vi "pp3_cam_display.vi"(8 "Camera":T1="cam0", 9 "Log File Directory":refnum<vi>, 10 "State info Refnum":refnum<vi>, 11 "Image Ctl Refnum":refnum<vi>) -> ()   [LabVIEW 2013]
doc: "This VI is a general VI that loops through webcam images, and saves when necessary. It should be run asynchronously, so that webcam display/logging is independent of the main loop. Terminate this VI by setting the \"Webcam on\" value within the state info refnum to False."
uses:
  pp3_CTL_StateInfo.ctl
  pp3_CTL_State.ctl
  pp3_CTL_Trial.ctl
  pp3_CTL_TrialType.ctl
  labolabo2/waveforms/WFTypes.ctl
  <vilib>/userdefined/High Color/IMAQdx.ctl
  <vilib>/vision/Image Controls.llb/IMAQ Image.ctl
  <vilib>/vision/driver/NI_Vision_Acquisition_Software.lvlib
panel:
  out "error out":errorcluster
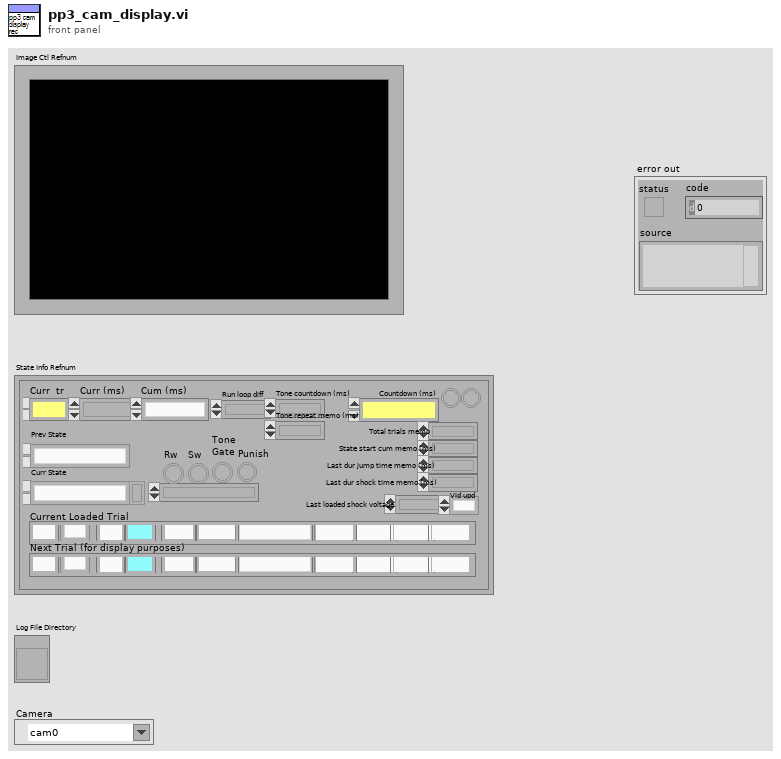
[diagram p1: front panel]
types:
  T1 = typedef "IMAQdx.ctl" = refnum<k21>
  T2 = typedef "pp3_CTL_StateInfo.ctl" = cluster{"Curr  tr":u16, "Curr (ms)":u32, "Cum (ms)":i64, "Run loop diff":i64, "Tone countdown (ms)":i64, "Countdown (ms)":i64, "Curr State":T3, "Prev State":T3, "Rw":bool, "Sw":bool, "Tone\nGate":bool, "Punish":bool, "Current DAQ DO Int":u16, "Current Loaded Trial":T4, "Next Trial (for display purposes)":T4, "Total trials memo":i64, "State start cum memo (ms)":i64, "Last dur jump time memo (ms)":i64, "Last dur shock time memo (ms)":i64, "Tone repeat memo (ms)":i64, "Webcam on":bool, "Webcam recording":bool, "State update flag":bool, "Last loaded shock voltage":dbl, "Vid upd":enum16{"0", "1", "2", "3", "4", "5", "6", "7", "8", "9"}}
  T3 = typedef "pp3_CTL_State.ctl" = enum8{"0 NULL", "1 Habituation", "2 (Load Trial)", "3 Stay Period", "4 Load Audio/Click Delay", "5 GO Trial", "6 GO Jumped", "7 GO Timeout", "8 NOGO Trial", "9 NOGO Jumped", "10 NOGO Timeout", "11 TEST Trial", "12 TEST Jumped", "13 TEST Timeout", "14 Intertrial Interval", "15 Done"}
  T4 = typedef "pp3_CTL_Trial.ctl" = cluster{"Trial Type Number":i16, "Trial Type":T5, "Trial Weight":u32, "Shock (mA)":dbl, "Duration (ms)":dbl, "Sound Type":T6, "Stim P1":dbl, "Stim P2":dbl, "Stim P3":dbl, "Stim P4":dbl, "DAQ Amplitude (V)":dbl}
  T5 = typedef "pp3_CTL_TrialType.ctl" = enum16{"OFF", "GO", "NOGO", "TEST"}
  T6 = typedef "WFTypes.ctl" = enum16{"00 NULL", "01 DC", "02 Noise", "03 Pure Tone", "04 FM Sweep"}
  T7 = typedef "IMAQ Image.ctl" = refnum<image>
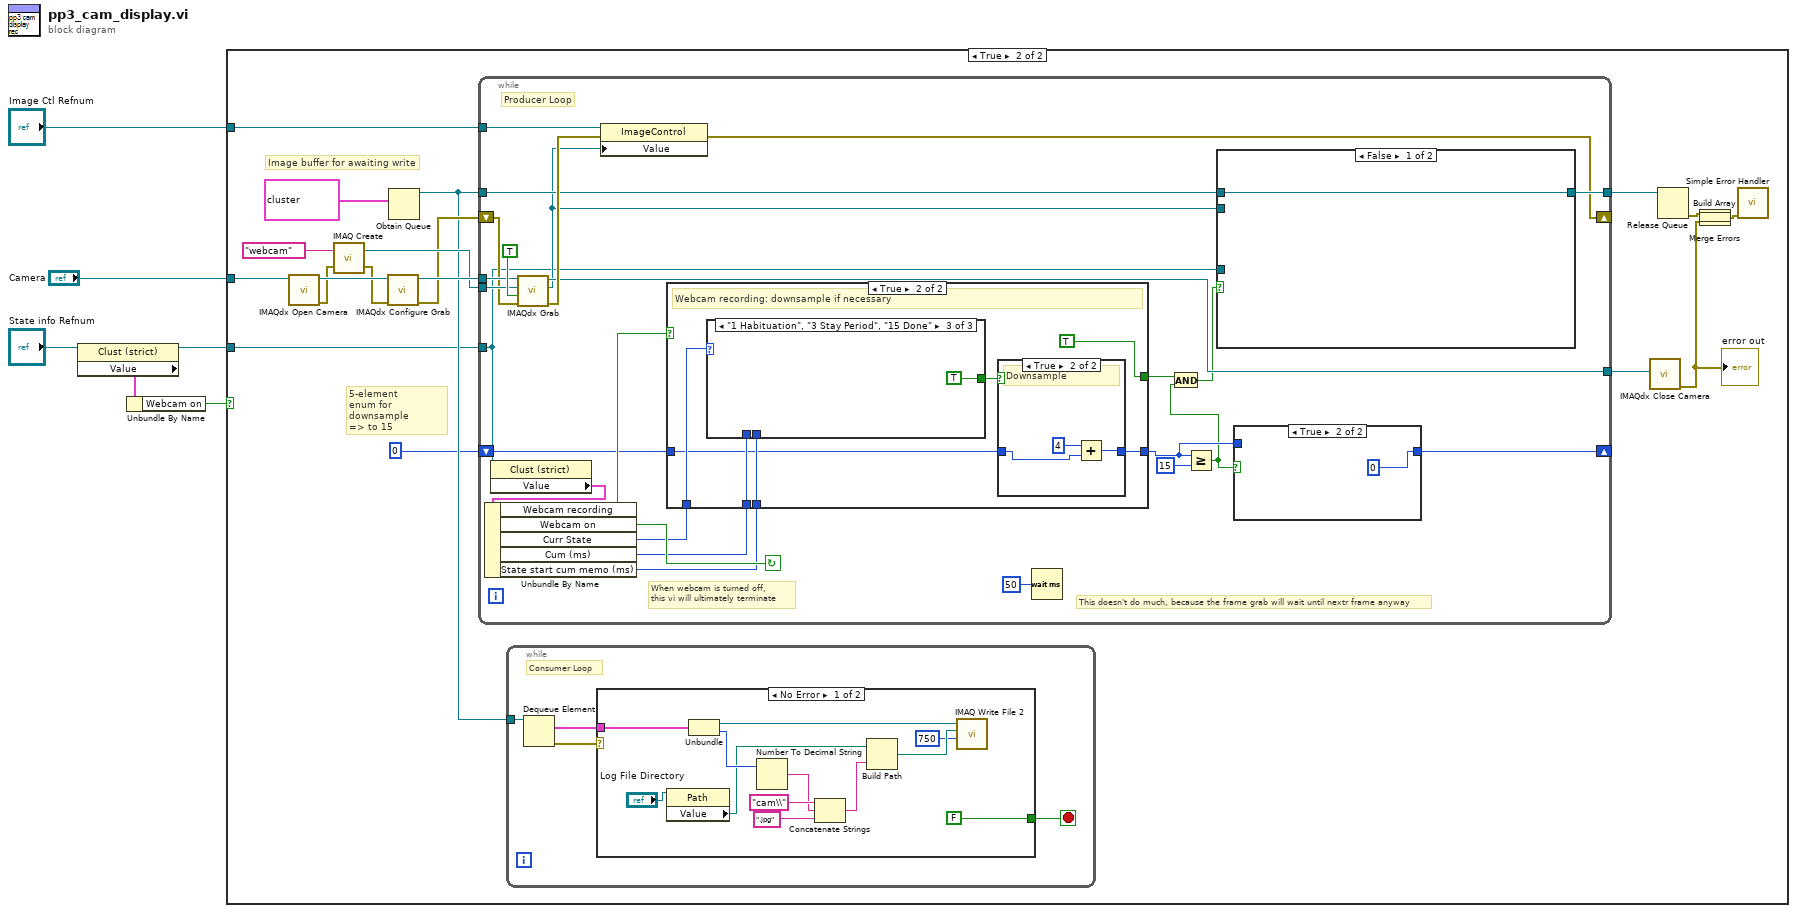
[diagram p0: block diagram]
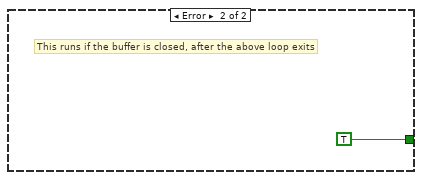
[diagram p3: hidden frame]
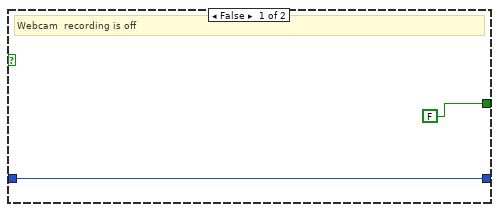
[diagram p5: hidden frame]
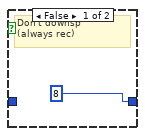
[diagram p6: hidden frame]
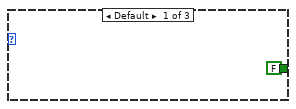
[diagram p7: hidden frame]
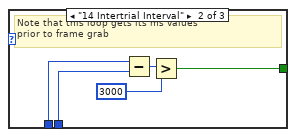
[diagram p8: hidden frame]
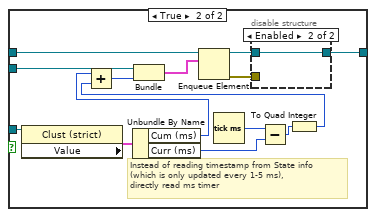
[diagram p9: hidden frame]
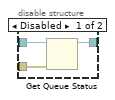
[diagram p10: hidden frame]
diagram:
  n1 = property class="Clust (strict)"(reference="State info Refnum") -> (reference out=w3:refnum<vi>, "Value"=w2:T2)  [unwired: 1 in, 1 out]
  n2 = Unbundle By Name(w2) -> ("Webcam on"=w1:bool)
  n3 = case shown="True" w1 {
    tunnel: "Image Ctl Refnum" -> [_ w25]
    tunnel: "Camera" -> [_ w21]
    tunnel: w3 -> [_ w8]
    frame False {
    }
    frame True {
      # "5-element\nenum for downsample\n=> to 15"
      # "Image buffer for awaiting write"
      n4 = call <vilib>:"IMAQdx Open Camera.vi"("Session In"=w21) -> ("error out"=w20:errorcluster, "Session Out"=w23:T1)  [unwired: 9 in]
      n5 = call "IMAQ Create"("Image Name"="webcam", "error in (no error)"=w20) -> ("New Image"=w17:T7, "error out"=w19:errorcluster)  [unwired: 3 in]
      n6 = call <vilib>:"IMAQdx Configure Grab.vi"("error in"=w19, "Session In"=w23) -> ("error out"=w11:errorcluster, "Session Out"=w18:T1)  [unwired: 8 in]
      n7 = Obtain Queue(element data type=cluster{"Image":T7, "Cum (ms)":i64} {"Image"="Webcam", "Cum (ms)"=0}) -> (queue out=w9:refnum<queue>)  [unwired: 4 in, 2 out]
      n8 = while {
        tunnel: w18 -> [w65]
        tunnel: w17 -> [w64]
        tunnel: w9 -> [w63]
        tunnel: [w61] -> w16
        tunnel: [w60] -> w12
        shift-right: [w57] -> _
        shift-left: w11 -> [w59]
        tunnel: w8 -> [w56]
        tunnel: w25 -> [w67]
        shift-right: [w48] -> _
        shift-left: 0 -> [w50]
        stop <- w62 continue-if-true
        # "This doesn't do much, because the frame grab will wait until nextr frame anyway"
        # "When webcam is turned off,\nthis vi will ultimately terminate"
        # "Producer Loop"
        n9 = property class="Clust (strict)"(reference=w56) -> ("Value"=w54:T2)  [unwired: 1 in, 2 out]
        n10 = Unbundle By Name(w54) -> ("Webcam recording"=w55:bool, "Webcam on"=w62:bool, "Curr State"=w53:T3, "Cum (ms)"=w52:i64, "State start cum memo (ms)"=w51:i64)
        n11 = call <vilib>:"IMAQdx Grab.vi"("error in"=w59, "Wait for Next Buffer? (Yes)"=TRUE, "Image In"=w64, "Session In"=w65) -> ("error out"=w68:errorcluster, "Image Out"=w58:T7, "Session Out"=w61:T1)  [unwired: 4 in, 1 out]
        n12 = property class="ImageControl"(reference=w67, error in=w68, "Value"=w58) -> (error out=w57:errorcluster)  [unwired: 1 out]
        n13 = case shown="True" w55 {
          tunnel: [w72 w78] -> w47
          tunnel: w53 -> [_ w77]
          tunnel: w52 -> [_ w76]
          tunnel: w51 -> [_ w75]
          tunnel: w50 -> [w72 w74]
          tunnel: [FALSE TRUE] -> w44
          frame False {
            # "Webcam  recording is off"
          }
          frame True {
            # "Webcam recording: downsample if necessary"
            n14 = case shown="\"1 Habituation\", \"3 Stay Period\", \"15 Done\"" w77 {
              tunnel: [FALSE w87 TRUE] -> w79
              tunnel: w76 -> [_ w86 _]
              tunnel: w75 -> [_ w85 _]
              frame Default {
              }
              frame "14 Intertrial Interval" {
                # "Note that this loop gets its ms values\nprior to frame grab"
                n15 = Subtract(x=w86, y=w85) -> (x-y=w89:i64)
                n16 = Greater?(x=w89, y=i64 3000) -> (0:w87:bool)
              }
              frame "1 Habituation", "3 Stay Period", "15 Done" {
              }
            }
            n17 = case shown="True" w79 {
              tunnel: [8 ("x") w81] -> w78
              tunnel: w74 -> [_ w82]
              frame False {
                # "Don't downsp\n(always rec)"
              }
              frame True {
                # "Downsample"
                n18 = Add(x=4, y=w82) -> (x+y=w81:i32)
              }
            }
          }
        }
        n19 = Wait (ms)(milliseconds to wait=u32 50) -> ()  [unwired: 1 out]
        n20 = Greater Or Equal?(x=w47, y=15) -> (x >= y?=w45:bool)
        n21 = And(x=w44, y=w45) -> (x .and. y?=w46:bool)
        n22 = case shown="False" w46 {
          tunnel: w58 -> [_ w105]
          tunnel: w63 -> [w91 w104]
          tunnel: [w91 w102] -> w60
          tunnel: w56 -> [_ w99]
          frame False {
          }
          frame True {
            # "Instead of reading timestamp from State info\n(which is only updated every 1-5 ms), \ndirectly read ms timer"
            n23 = property class="Clust (strict)"(reference=w99) -> ("Value"=w98:T2)  [unwired: 1 in, 2 out]
            n24 = Unbundle By Name(w98) -> ("Cum (ms)"=w93:i64, "Curr (ms)"=w97:u32)
            n25 = Tick Count (ms)() -> (millisecond timer value=w100:u32)
            n26 = Subtract(x=w100, y=w97) -> (x-y=w95:u32)
            n27 = To Quad Integer(1:w95) -> (0:w94:i64)
            n28 = Add(x=w93, y=w94) -> (x+y=w92:i64)
            n29 = Bundle("Image Out"=w105, w92) -> (w96:cluster{"Image Out":T7, i64})  [unwired: 1 in]
            n30 = Enqueue Element(queue=w104, element=w96) -> (queue out=w103:refnum<queue>, error out=w101:errorcluster)  [unwired: 2 in, 1 out]
            n31 = disable-structure shown="Enabled" {
              disable-tunnel: w103 -> [w108 w109]
              disable-tunnel: [w107 w109] -> w102
              disable-tunnel: w101 -> [w106 _]
              frame Disabled {
                n32 = Get Queue Status(queue=w108, error in (no error)=w106) -> (queue out=w107:refnum<queue>)  [unwired: 1 in, 7 out]
              }
              frame Enabled {
              }
            }
          }
        }
        n33 = case shown="True" w45 {
          tunnel: [w69 0 ("y")] -> w48
          tunnel: w47 -> [w69 _]
          frame False {
          }
          frame True {
          }
        }
      }
      n34 = while {
        tunnel: w9 -> [w29]
        stop <- w27 stop-if-true
        # "Consumer Loop"
        n35 = Dequeue Element(queue=w29) -> (element=w26:cluster{"Image":T7, "Cum (ms)":i64}, error out=w28:errorcluster)  [unwired: 2 in, 2 out]
        n36 = case shown="No Error" w28 {
          tunnel: [FALSE TRUE] -> w27
          tunnel: w26 -> [w40 _]
          frame No Error {
            n37 = property class="Path"(reference="Log File Directory") -> ("Value"=w31:path)  [unwired: 1 in, 2 out]
            n38 = Unbundle(w40) -> ("Image"=w33:T7, "Cum (ms)"=w37:i64)
            n39 = Number To Decimal String(number=w37) -> (decimal integer string=w36:string)  [unwired: 1 in]
            n40 = Concatenate Strings("cam\\", w36, ".jpg" ("string")) -> (w35:string)
            n41 = Build Path(base path=w31, name or relative path=w35) -> (appended path=w34:path)
            n42 = call-poly "IMAQ Write File 2"("Image Quality"=u32 750, "File Path"=w34, "Image"=w33) -> ()  [unwired: 7 in, 2 out]
          }
          frame Error {
            # "This runs if the buffer is closed, after the above loop exits"
          }
        }
      }
      n43 = call <vilib>:"IMAQdx Close Camera.vi"("Session In"=w16) -> ("error out"=w10:errorcluster)  [unwired: 10 in]
      "error out" <- w10
      n44 = Release Queue(queue=w12) -> (error out=w15:errorcluster)  [unwired: 2 in, 2 out]
      n45 = Build Array(w15, w10) -> (w13:errorcluster[])
      n46 = Merge Errors(w13) -> (w14:errorcluster)
      n47 = call <vilib>:"Simple Error Handler.vi"("error in (no error)"=w14) -> ()  [unwired: 4 in, 5 out]
    }
  }
